vi "StartData.vi"(8 "error in (no error)":errorcluster, 11 "Class In":refnum<class "C37.118 PMU.lvclass">) -> (0 "error out":errorcluster, 3 "Class Out":refnum<class "C37.118 PMU.lvclass">)   [LabVIEW 2018, in "SensorPlugins.lvlib" / "C37.118 PMU.lvclass"]
uses:
  C37.118 PMU.lvclass
  C37.118 PMU.lvclass/C37.118 PMU.ctl
  Typedef/eCmdTypes.ctl
  <userlib>/NIST/Socket Class/Classes/Socket.Base/Socket.Base.lvclass/Socket.Base.ctl
  <userlib>/NIST/Socket Class/Classes/Socket.Base/Accessors/Read connected.vi
  Accessors/Read CmdSocket.vi
  Accessors/Read PMUComms.vi
  Accessors/Read DataSocket.vi
  Accessors/Write CmdSocket.vi
  Accessors/Write DataSocket.vi
  Accessors/Read PMUConfigData.vi
  <userlib>/NIST/Socket Class/Classes/Socket.Base/Socket.Base.lvclass
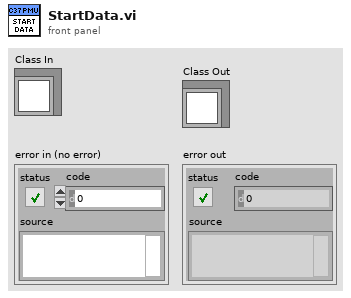
[diagram p1: front panel]
types:
  T1 = typedef "SensorPlugins.lvlib/C37.118 PMU.lvclass/eCmdTypes.ctl" = enum16{"Stop realtime data", "Start realtime data", "Send HDR file", "Send CFG-1 file", "Send CFG-2 file"}
  T2 = typedef "SensorPlugins.lvlib/C37.118 PMU.lvclass/PMUConfigData.ctl" = cluster{"TimeBase":u32, "NUM_PMU":u16, "Station Name":string, "IDCODE":u16, "PHRNMR":u16, "ANNMR":u16, "DIGNMR":u16, "FORMAT BITS":T3, "Valid Inputs":u16[], "DigitalStatusMask":u16[], "24bit_PHUNIT":i32[], "24bit_ANUNIT":u32[], "Analog Amplitude Setting":u32[], "Unit (Vor I)":u8[], "ChannelNames":string, "Fs":i16, "SOC ":u32, "FRACSEC":u32, "F0":sgl, "CFGCNT":u16}
  T3 = typedef "SensorPlugins.lvlib/C37.118 PMU.lvclass/FormatBits.ctl" = cluster{"Rect/Polar":bool, "Phasor Int/Float":bool, "Analog Int/Float":bool, "F/ROCOF Int/Float":bool}
  T4 = typedef "SensorPlugins.lvlib/C37.118 PMU.lvclass/PMUComms.ctl" = cluster{"PMU IP Address":string, "CMD Comms Type":T5, "Data Comms Type":T5, "CMD Port":u16, "Data Port":u16, "PMU ID":u16}
  T5 = typedef "SensorPlugins.lvlib/C37.118 PMU.lvclass/eCommsType.ctl" = enum16{"TCP", "UDP", "USB", "GPIB"}
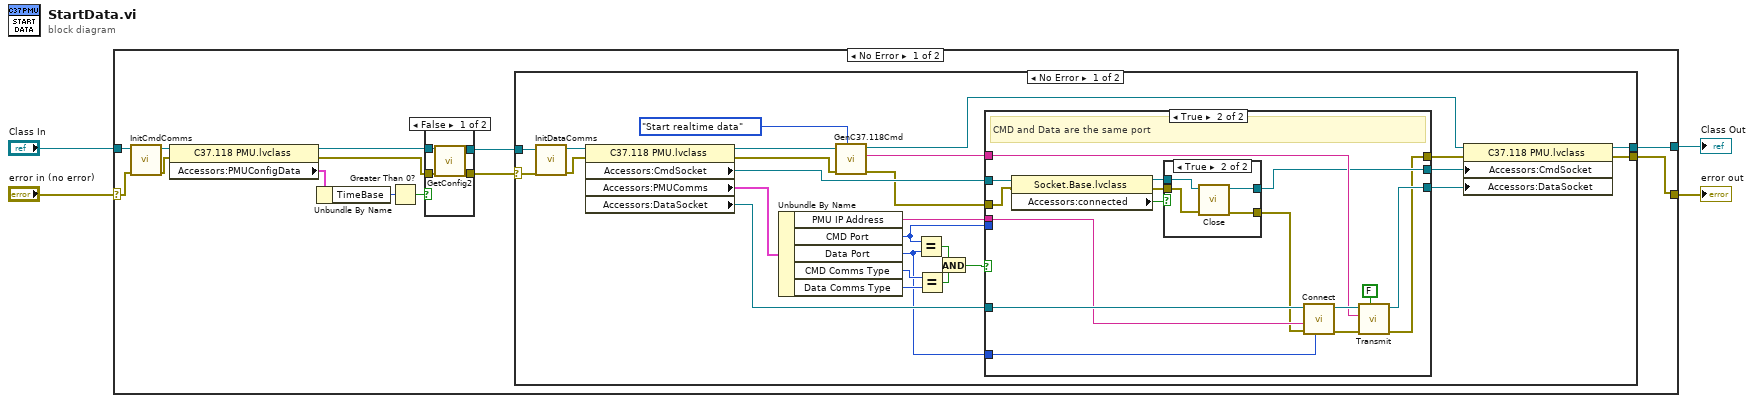
[diagram p0: block diagram]
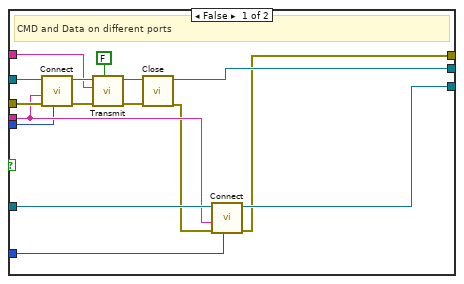
[diagram p2: hidden frame]
diagram:
  n1 = case shown="No Error" "error in (no error)" {
    selector: "error in (no error)" -> [w16 w90]
    tunnel: "Class In" -> [w17 w91]
    tunnel: [w14 w91] -> w2
    tunnel: [w13 w90] -> w1
    frame No Error {
      n2 = call "InitCmdComms.vi"("error in (no error)"=w16, "C37.118 PMU in"=w17) -> ("error out"=w7:errorcluster, "C37.118 PMU out"=w15:refnum<class "C37.118 PMU.lvclass">)  [unwired: 8 in]
      n3 = property class="C37.118 PMU.lvclass"(reference=w15, error in=w7) -> (reference out=w10:refnum<class "C37.118 PMU.lvclass">, error out=w6:errorcluster, "Accessors:PMUConfigData"=w12:T2)
      n4 = Unbundle By Name(w12) -> ("TimeBase"=w9:u32)
      n5 = Greater Than 0?(x=w9) -> (x > 0?=w8:bool)
      n6 = case shown="False" w8 {
        tunnel: [w87 w89] -> w11
        tunnel: w10 -> [w86 w89]
        tunnel: w6 -> [w85 w88]
        tunnel: [w84 w88] -> w5
        frame False {
          n7 = call "GetConfig2.vi"("error in (no error)"=w85, "C37.118 PMU in"=w86) -> ("error out"=w84:errorcluster, "C37.118 PMU out"=w87:refnum<class "C37.118 PMU.lvclass">)  [unwired: 8 in]
        }
        frame True {
        }
      }
      n8 = case shown="No Error" w5 {
        selector: w5 -> [w18 w82]
        tunnel: [w35 w83] -> w14
        tunnel: [w30 w82] -> w13
        tunnel: w11 -> [w19 w83]
        frame No Error {
          n9 = call "InitDataComms.vi"("error in (no error)"=w18, "C37.118 PMU in"=w19) -> ("error out"=w36:errorcluster, "C37.118 PMU out"=w37:refnum<class "C37.118 PMU.lvclass">)  [unwired: 8 in]
          n10 = property class="C37.118 PMU.lvclass"(reference=w37, error in=w36) -> (reference out=w42:refnum<class "C37.118 PMU.lvclass">, error out=w32:errorcluster, "Accessors:CmdSocket"=w41:refnum<class "Socket.Base.lvclass">, "Accessors:PMUComms"=w40:T4, "Accessors:DataSocket"=w33:refnum<class "Socket.Base.lvclass">)
          n11 = Unbundle By Name(w40) -> ("PMU IP Address"=w31:string, "CMD Port"=w22:u16, "Data Port"=w21:u16, "CMD Comms Type"=w27:T5, "Data Comms Type"=w26:T5)
          n12 = call "GenC37.118Cmd.vi"("Function"=eCmdTypes."Start realtime data", "error in (no error)"=w32, "PMUClass"=w42) -> ("error out"=w38:errorcluster, "Command"=w39:string, "PMUClass"=w20:refnum<class "C37.118 PMU.lvclass">)  [unwired: 6 in]
          n13 = Equal?(x=w22, y=w21) -> (x = y?=w25:bool)
          n14 = Equal?(x=w27, y=w26) -> (x = y?=w24:bool)
          n15 = And(x=w25, y=w24) -> (x .and. y?=w23:bool)
          n16 = case shown="True" w23 {
            tunnel: w41 -> [w59 w69]
            tunnel: w39 -> [w55 w70]
            tunnel: w38 -> [w54 w68]
            tunnel: [w51 w64] -> w34
            tunnel: w33 -> [w50 w75]
            tunnel: w31 -> [w49 w73]
            tunnel: [w48 w61] -> w29
            tunnel: [w46 w60] -> w28
            tunnel: w22 -> [w45 _]
            tunnel: w21 -> [w44 w74]
            frame False {
              # "CMD and Data on different ports"
              n17 = call-dynamic "Connect.vi"("remote_port"=w45, "error in (no error)"=w54, "remote_address"=w49, "Socket.Base in"=w59) -> ("error out"=w56:errorcluster, "Socket.Base out"=w57:refnum<class "Socket.Base.lvclass">)  [unwired: 6 in]
              n18 = call-dynamic "Transmit.vi"("packet? (f)"=FALSE, "error in (no error)"=w56, "data"=w55, "Socket.Base in"=w57) -> ("error out"=w53:errorcluster, "Socket.Base out"=w52:refnum<class "Socket.Base.lvclass">)  [unwired: 5 in, 1 out]
              n19 = call-dynamic "Close.vi"("error in (no error)"=w53, "Socket.Base in"=w52) -> ("error out"=w47:errorcluster, "Socket.Base out"=w51:refnum<class "Socket.Base.lvclass">)  [unwired: 8 in]
              n20 = call-dynamic "Connect.vi"("remote_port"=w44, "error in (no error)"=w47, "remote_address"=w49, "Socket.Base in"=w50) -> ("error out"=w46:errorcluster, "Socket.Base out"=w48:refnum<class "Socket.Base.lvclass">)  [unwired: 6 in]
            }
            frame True {
              # "CMD and Data are the same port"
              n21 = property class="Socket.Base.lvclass"(reference=w69, error in=w68) -> (reference out=w66:refnum<class "Socket.Base.lvclass">, error out=w65:errorcluster, "Accessors:connected"=w67:bool)
              n22 = case shown="True" w67 {
                tunnel: w66 -> [w77 w81]
                tunnel: w65 -> [w76 w80]
                tunnel: [w76 w79] -> w63
                tunnel: [w77 w78] -> w64
                frame False {
                }
                frame True {
                  n23 = call-dynamic "Close.vi"("error in (no error)"=w80, "Socket.Base in"=w81) -> ("error out"=w79:errorcluster, "Socket.Base out"=w78:refnum<class "Socket.Base.lvclass">)  [unwired: 8 in]
                }
              }
              n24 = call-dynamic "Connect.vi"("remote_port"=w74, "error in (no error)"=w63, "remote_address"=w73, "Socket.Base in"=w75) -> ("error out"=w72:errorcluster, "Socket.Base out"=w71:refnum<class "Socket.Base.lvclass">)  [unwired: 6 in]
              n25 = call-dynamic "Transmit.vi"("packet? (f)"=FALSE, "error in (no error)"=w72, "data"=w70, "Socket.Base in"=w71) -> ("error out"=w60:errorcluster, "Socket.Base out"=w61:refnum<class "Socket.Base.lvclass">)  [unwired: 5 in, 1 out]
            }
          }
          n26 = property class="C37.118 PMU.lvclass"(reference=w20, error in=w28, "Accessors:CmdSocket"=w34, "Accessors:DataSocket"=w29) -> (reference out=w35:refnum<class "C37.118 PMU.lvclass">, error out=w30:errorcluster)
        }
        frame Error {
        }
      }
    }
    frame Error {
    }
  }
  "Class Out" <- w2
  "error out" <- w1
